vi "IdentifierCodefromVIdeo.vi"() -> ()   [LabVIEW 2016]
uses:
  <vilib>/NXT/Block Support/NXT_InputPort.ctl
  <vilib>/NXT/Dual Mode Library/Waits/Wait_Bump.vi
  <vilib>/NXT/Dual Mode Library/Sensors/Touch_Pressed.vi
  <vilib>/NXT/Dual Mode Library/Sensors/EV3_Color_RGB.vi
  <vilib>/NXT/Dual Mode Library/prims/inRangeAndCoerce/inRangeAndCoerce_int.vi
  <vilib>/NXT/Dual Mode Library/Sensors/EV3_Color_Color.vi
panel:
  out "Color Size\n  Output 9":string
  out "Color Size\n  Output 8":string
  out "Color Size\n  Output 7":string
  out "Color Size\n  Output":string
  out "Color Size\n  Output 6":string
  out "Color Size\n  Output 4":string
  out "Color Size\n  Output 3":string
  out "Color Size\n  Output 2":string
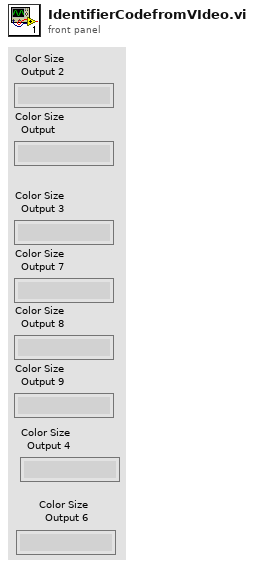
[diagram p1: front panel]
types:
  T1 = typedef "NXT_InputPort.ctl" = u32
  T2 = typedef "LVHSConnector.ctl" = refnum<class "BrickReference.lvclass">
  T3 = typedef "ColorSensorColors.ctl" = enum16{"No Color", "Black", "Blue", "Green", "Yellow", "Red", "White", "Brown"}
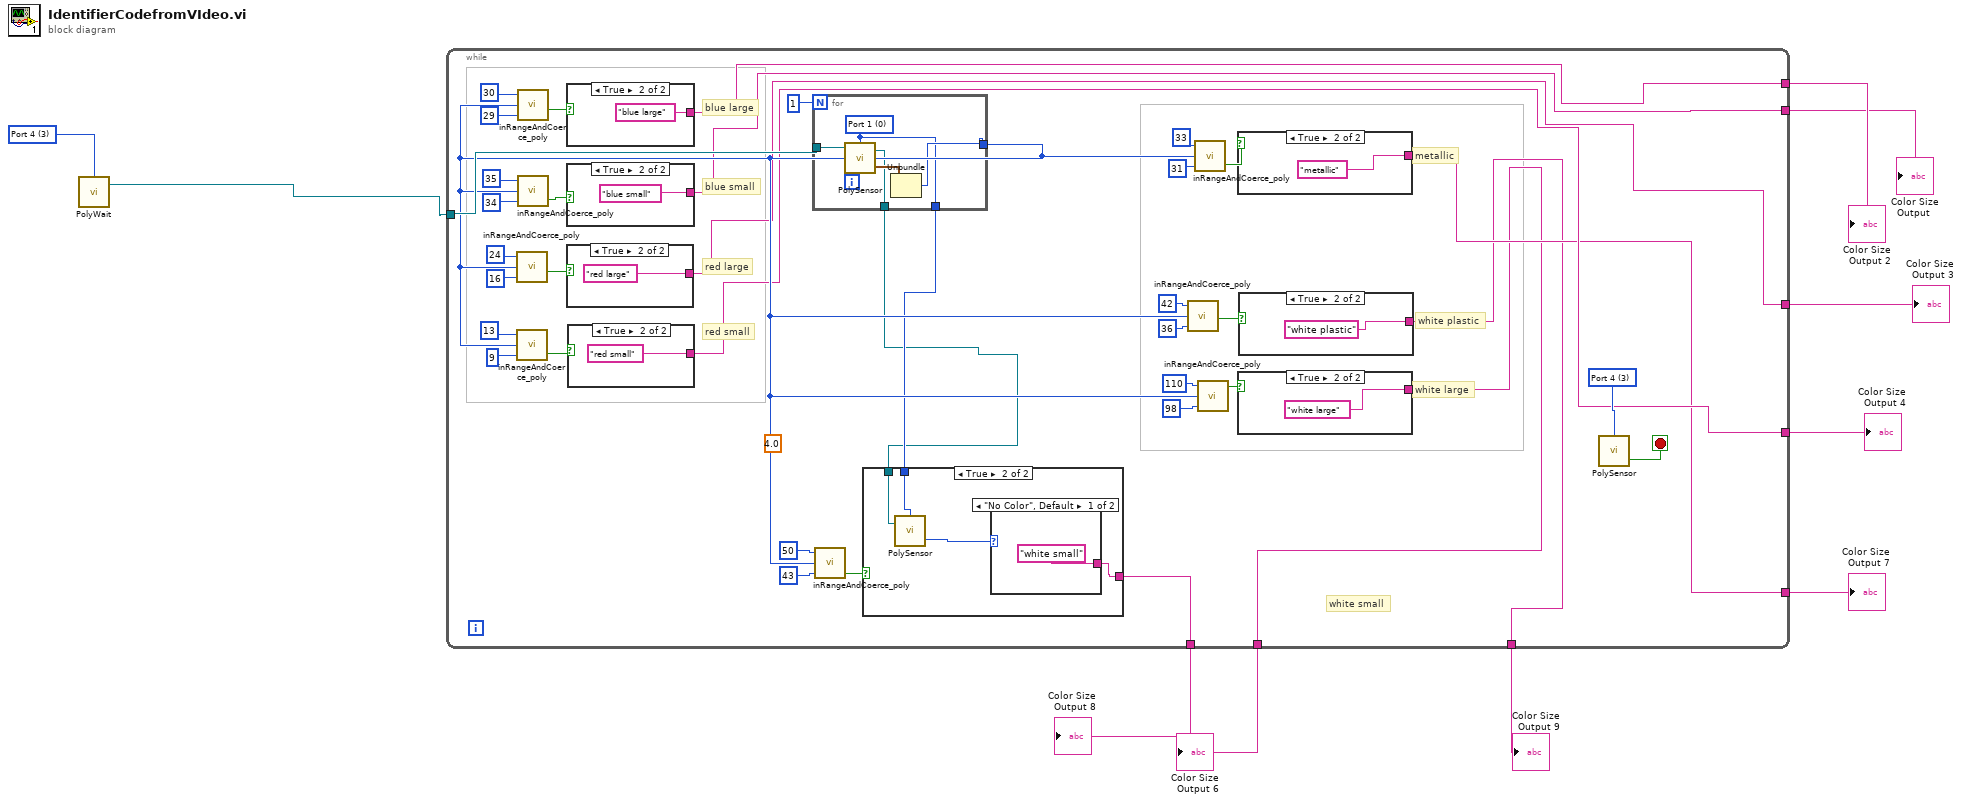
[diagram p0: block diagram]
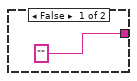
[diagram p2: hidden frame]
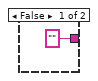
[diagram p3: hidden frame]
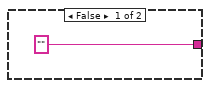
[diagram p4: hidden frame]
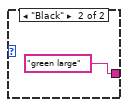
[diagram p5: hidden frame]
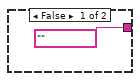
[diagram p6: hidden frame]
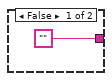
[diagram p7: hidden frame]
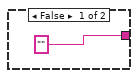
[diagram p8: hidden frame]
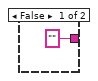
[diagram p9: hidden frame]
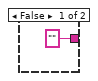
[diagram p10: hidden frame]
diagram:
  w9 = T1 3 items=["Port 1", "Port 2", "Port 3", "Port 4"] ("Port (Port 1)")
  n1 = call-poly <vilib>:"PolyWait.vi"("Port (Port 1)"=w9) -> ("NXT/EV3"=w10:T2)  [unwired: 3 in]
  n2 = while {
    tunnel: w10 -> [w25]
    tunnel: [w19] -> w8
    tunnel: [w18] -> w7
    tunnel: [w17] -> w6
    tunnel: [w16] -> w5
    tunnel: [w15] -> w4
    tunnel: [w14] -> w3
    tunnel: [w13] -> w2
    tunnel: [w12] -> w1
    stop <- w28 stop-if-true
    (unwired) sgl 4.0 ("Time (1 sec)")
    w27 = T1 3 items=["Port 1", "Port 2", "Port 3", "Port 4"] ("Port (Port 1)")
    # "metallic"
    # "white plastic"
    # "white small"
    # "white large"
    # "red small"
    # "red large"
    # "blue small"
    # "blue large"
    n3 = for {
      N: 1 -> [_]
      tunnel: w25 -> [w53]
      tunnel: [w52] -> w21
      tunnel: [w51] -> w11
      tunnel: [w50] -> w20
      w50 = T1 0 items=["Port 1", "Port 2", "Port 3", "Port 4"] ("Port (Port 1)")
      n4 = call-poly <vilib>:"PolySensor.vi"("NXT/EV3"=w53, "Port (Port 1)"=w50) -> ("RGB Color"=w54:cluster{"Red":u8, "Green":u8, "Blue":u8}, "NXT/EV3"=w51:T2)  [unwired: 1 in]
      n5 = Unbundle(w54) -> ("Green"=w52:u8)  [unwired: 2 out]
    }
    n6 = call-poly <vilib>:"inRangeAndCoerce_poly.vi"("lower limit"=16, "x"=w21, "upper limit"=24) -> ("In Range?"=w34:bool)  [unwired: 1 out]
    n7 = call-poly <vilib>:"inRangeAndCoerce_poly.vi"("lower limit"=9, "x"=w21, "upper limit"=13) -> ("In Range?"=w33:bool)  [unwired: 1 out]
    n8 = call-poly <vilib>:"inRangeAndCoerce_poly.vi"("lower limit"=29, "x"=w21, "upper limit"=30) -> ("In Range?"=w36:bool)  [unwired: 1 out]
    n9 = call-poly <vilib>:"inRangeAndCoerce_poly.vi"("lower limit"=34, "x"=w21, "upper limit"=35) -> ("In Range?"=w35:bool)  [unwired: 1 out]
    n10 = case shown="True" w36 {
      tunnel: ["" "blue large"] -> w19
      frame False {
      }
      frame True {
      }
    }
    n11 = case shown="True" w35 {
      tunnel: ["" "blue small"] -> w18
      frame False {
      }
      frame True {
      }
    }
    n12 = case shown="True" w34 {
      tunnel: ["" "red large"] -> w17
      frame False {
      }
      frame True {
      }
    }
    n13 = case shown="True" w33 {
      tunnel: ["" "red small"] -> w16
      frame False {
      }
      frame True {
      }
    }
    n14 = call-poly <vilib>:"inRangeAndCoerce_poly.vi"("lower limit"=43, "x"=w21, "upper limit"=50) -> ("In Range?"=w31:bool)  [unwired: 1 out]
    n15 = case shown="True" w31 {
      tunnel: ["" w61] -> w13
      tunnel: w20 -> [_ w63]
      tunnel: w11 -> [_ w60]
      frame False {
      }
      frame True {
        n16 = call-poly <vilib>:"PolySensor.vi"("NXT/EV3"=w60, "Port (Port 1)"=w63) -> ("Detected Color"=w62:T3)  [unwired: 1 in, 1 out]
        n17 = case shown="\"No Color\", Default" w62 {
          tunnel: ["white small" "green large"] -> w61
          frame "No Color", Default {
          }
          frame "Black" {
          }
        }
      }
    }
    n18 = call-poly <vilib>:"inRangeAndCoerce_poly.vi"("lower limit"=36, "x"=w21, "upper limit"=42) -> ("In Range?"=w30:bool)  [unwired: 1 out]
    n19 = call-poly <vilib>:"inRangeAndCoerce_poly.vi"("lower limit"=31, "x"=w21, "upper limit"=33) -> ("In Range?"=w22:bool)  [unwired: 1 out]
    n20 = call-poly <vilib>:"inRangeAndCoerce_poly.vi"("lower limit"=98, "x"=w21, "upper limit"=110) -> ("In Range?"=w32:bool)  [unwired: 1 out]
    n21 = case shown="True" w22 {
      tunnel: ["" "metallic"] -> w15
      frame False {
      }
      frame True {
      }
    }
    n22 = case shown="True" w32 {
      tunnel: ["" "white large"] -> w12
      frame False {
      }
      frame True {
      }
    }
    n23 = case shown="True" w30 {
      tunnel: ["" "white plastic"] -> w14
      frame False {
      }
      frame True {
      }
    }
    n24 = call-poly <vilib>:"PolySensor.vi"("Port (Port 1)"=w27) -> ("Yes / No"=w28:bool)  [unwired: 2 in, 1 out]
  }
  "Color Size\n  Output 2" <- w8
  "Color Size\n  Output 3" <- w6
  "Color Size\n  Output" <- w7
  "Color Size\n  Output 9" <- w3
  "Color Size\n  Output 7" <- w4
  "Color Size\n  Output 4" <- w5
  "Color Size\n  Output 8" <- w2
  "Color Size\n  Output 6" <- w1
